vi "Valvole sistema _.vi"(10 "% valvole linea":dbl[](array[numeric]), 11 "Indici valvole linea":i16[](array[numeric])) -> (3 "Array Valvole sistema out %":dbl[](array[numeric]))   [LabVIEW 2019]
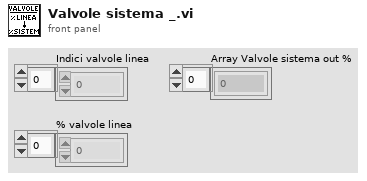
[diagram p1: front panel]
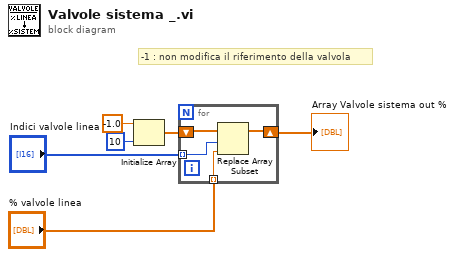
[diagram p0: block diagram]
diagram:
  # "-1 : non modifica il riferimento della valvola"
  n1 = Initialize Array(-1.0 ("element"), 10 ("dimension size")) -> (w1:dbl[])
  n2 = for {
    shift-right: [w9] -> w6
    shift-left: w1 -> [w10]
    tunnel: "Indici valvole linea" -> [w8] mode=indexing
    tunnel: "% valvole linea" -> [w7] mode=indexing
    n3 = Replace Array Subset(array=w10, new element=w7, index=w8) -> (w9:dbl[])
  }
  "Array Valvole sistema out %" <- w6
